vi "Initialize.vi"(7 "Serial Configuration":T1={"Baud Rate"=9600, "Parity"=0, "Data Bits"=8, "Stop Bits"=10, "Flow Control"=0} {"Flow Control" items=["None", "XON/XOFF", "RTS/CTS", "XON/XOFF & RTS/CTS", "DTR/DSR", "XON/XOFF & DTR/DSR"]; "Stop Bits" items=["1.0"=10, "1.5"=15, "2.0"=20]; "Data Bits" items=["7"=7, "8"=8]; "Parity" items=["None", "Odd", "Even", "Mark", "Space"]; "Baud Rate" items=["300"=300, "600"=600, "1200"=1200, "2400"=2400, "4800"=4800, "9600"=9600, "19200"=19200]}, 8 "error in":errorcluster, 9 "Reset":bool=TRUE, 10 "ID Query":bool=TRUE, 11 "VISA resource name":refnum<visa-resource-name>) -> (0 "error out":errorcluster, 3 "VISA resource name out":refnum<visa-resource-name>)   [LabVIEW 2020, in "IT-M3400.lvlib"]
doc: "Establishes communication with the instrument and optionally performs an instrument identification query and/or an instrument reset. It also places the instrument in a default state needed for other instrument driver operations. Therefore, call this VI before calling other instrument driver VIs for this instrument. Generally, you need to call the <b>Initialize</b> VI only once at the beginning of an application."
uses:
  IT-M3400.lvlib
panel:
  # "EDIT: Change control description to remove example text for buses not supported."
  # "EDIT: Serial settings must match those on the physical instrument.  Review user's manual to determine the correct Flow Control protocol for the instrument.  \"None\" is the least robust option for this setting, and could lead to unreliable data transmission."
  # "EDIT: If your instrument does not support ID query or Reset, remove the ID Query or Reset control from the front panel and delete the case structure with the ID Query or Reset code from the block diagram."
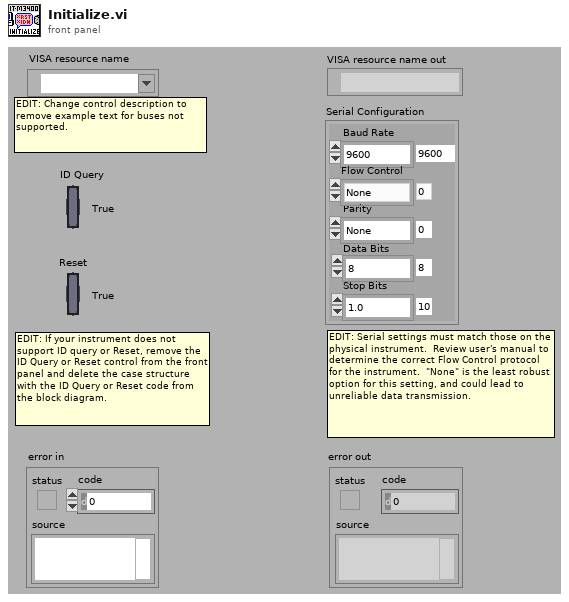
[diagram p1: front panel]
types:
  T1 = cluster{"Baud Rate":u32, "Parity":u16, "Data Bits":u16, "Stop Bits":u16, "Flow Control":u16}
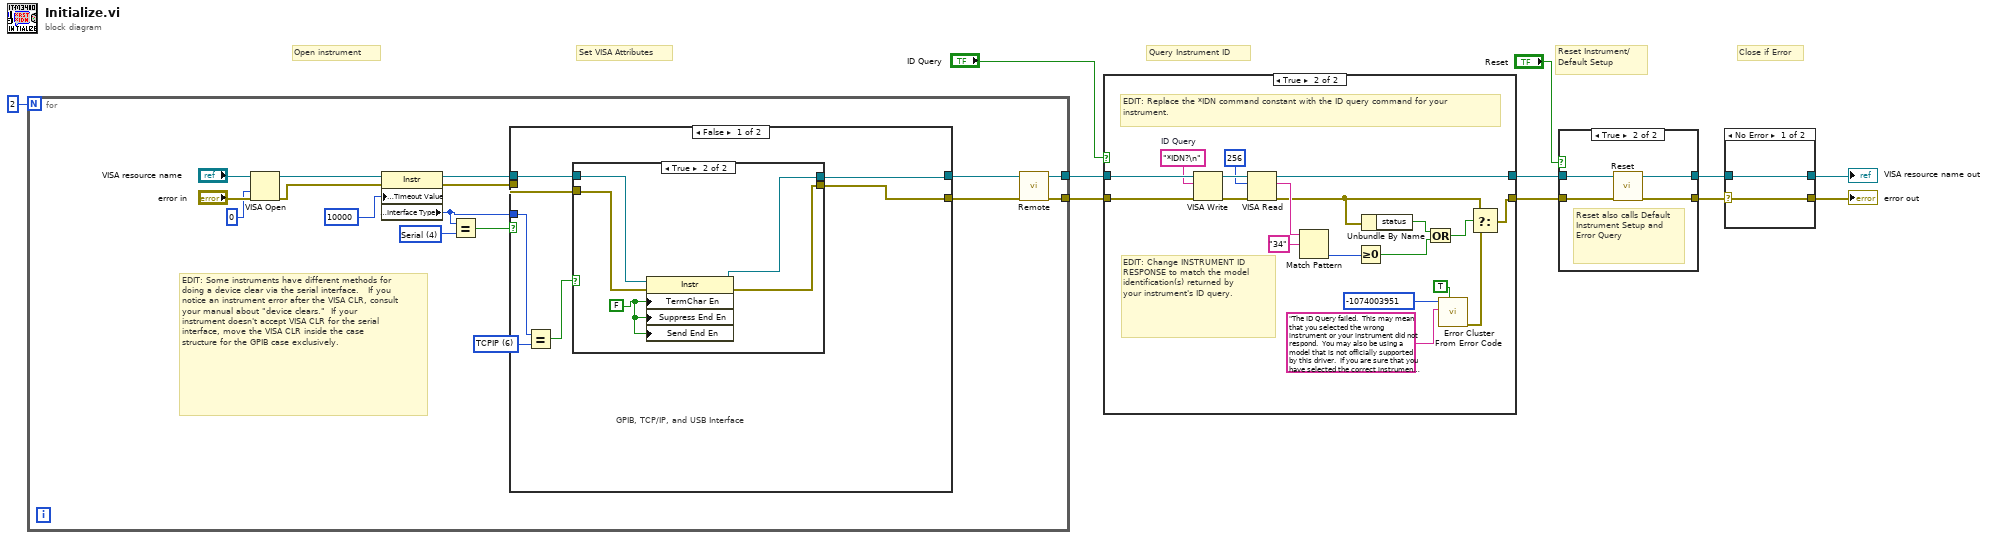
[diagram p0: block diagram]
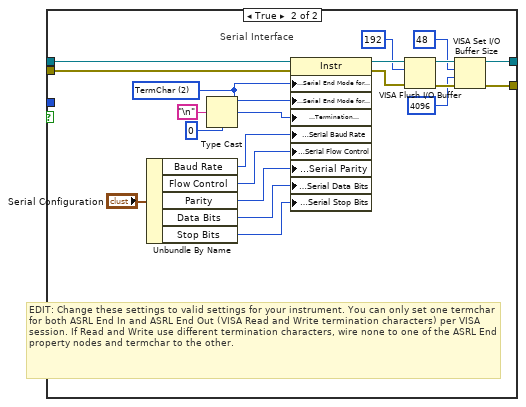
[diagram p3: hidden frame]
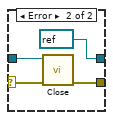
[diagram p4: hidden frame]
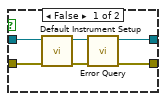
[diagram p5: hidden frame]
diagram:
  # "Set VISA Attributes"
  # "Close if Error"
  # "Query Instrument ID"
  # "Reset Instrument/\nDefault Setup"
  # "Open instrument"
  n1 = for {
    N: 2 -> [_]
    tunnel: [w16] -> w3
    tunnel: [w15] -> w2
    w21 = u16 4 items=["GPIB"=1, "VXI"=2, "GPIB-VXI"=3, "Serial"=4, "PXI"=5, "TCPIP"=6, "USB"=7] ("Interface Information:Interface Type")
    # "EDIT: Some instruments have different methods for doing a device clear via the serial interface.   If you notice an instrument error after the VISA CLR, consult your manual about \"device clears.\"  If your instrument doesn't accept VISA CLR for the serial interface, move the VISA CLR inside the case  structure for the GPIB case exclusively."
    n2 = VISA Open(access mode=u32 0, error in (no error)="error in", VISA resource name="VISA resource name") -> (VISA resource name=w13:refnum<visa-resource-name>, error out=w12:errorcluster)  [unwired: 2 in]
    n3 = property class="Instr"(reference=w13, error in=w12, "General Settings:Timeout Value"=u32 10000) -> (reference out=w23:refnum<visa-resource-name>, error out=w22:errorcluster, "Interface Information:Interface Type"=w19:u16)
    n4 = Equal?(x=w19, y=w21) -> (x = y?=w14:bool)
    n5 = case shown="False" w14 {
      tunnel: [w28 w58] -> w18
      tunnel: [w27 w55] -> w17
      tunnel: w23 -> [w30 w60]
      tunnel: w22 -> [w29 w61]
      tunnel: w19 -> [w31 _]
      frame False {
        w32 = u16 6 items=["GPIB"=1, "VXI"=2, "GPIB-VXI"=3, "Serial"=4, "PXI"=5, "TCPIP"=6, "USB"=7] ("Interface Information:Interface Type")
        # "GPIB, TCP/IP, and USB Interface"
        n6 = Equal?(x=w31, y=w32) -> (x = y?=w33:bool)
        n7 = case shown="True" w33 {
          tunnel: [w35 w40] -> w28
          tunnel: [w34 w39] -> w27
          tunnel: w30 -> [w35 w38]
          tunnel: w29 -> [w34 w37]
          frame False {
          }
          frame True {
            w36 = FALSE
            n8 = property class="Instr"(reference=w38, error in=w37, "TermChar En"=w36, "Suppress End En"=w36, "Send End En"=w36) -> (reference out=w40:refnum<visa-resource-name>, error out=w39:errorcluster)
          }
        }
      }
      frame True {
        w48 = u16 2 items=["None", "LastBit", "TermChar"] ("Serial Settings:Serial End Mode for Reads")
        # "EDIT: Change these settings to valid settings for your instrument. You can only set one termchar for both ASRL End In and ASRL End Out (VISA Read and Write termination characters) per VISA session. If Read and Write use different termination characters, wire none to one of the ASRL End property nodes and termchar to the other."
        # "Serial Interface"
        n9 = Unbundle By Name("Serial Configuration") -> ("Baud Rate"=w46:u32, "Flow Control"=w42:u16, "Parity"=w44:u16, "Data Bits"=w45:u16, "Stop Bits"=w41:u16)
        n10 = Type Cast(type=u8 0, x="\n" ("Line Feed Constant")) -> (*(type *) &x=w47:u8)
        n11 = property class="Instr"(reference=w60, error in=w61, "Serial Settings:Serial End Mode for Reads"=w48, "Serial Settings:Serial End Mode for Writes"=w48, "Message Based Settings:Termination Character"=w47, "Serial Settings:Serial Baud Rate"=w46, "Serial Settings:Serial Flow Control"=w42, "Serial Settings:Serial Parity"=w44, "Serial Settings:Serial Data Bits"=w45, "Serial Settings:Serial Stop Bits"=w41) -> (reference out=w54:refnum<visa-resource-name>, error out=w57:errorcluster)
        n12 = VISA Flush I/O Buffer(VISA resource name=w54, mask (16)=u16 192, error in (no error)=w57) -> (VISA resource name out=w59:refnum<visa-resource-name>, error out=w56:errorcluster)
        n13 = VISA Set I/O Buffer Size(VISA resource name=w59, mask (16)=u16 48, size (4096)=u32 4096 ("size (0)"), error in (no error)=w56) -> (VISA resource name out=w58:refnum<visa-resource-name>, error out=w55:errorcluster)
      }
    }
    n14 = call "Remote.vi"("error in"=w17, "VISA resource name"=w18) -> ("error out"=w15:errorcluster, "VISA resource name out"=w16:refnum<visa-resource-name>)  [unwired: 8 in]
  }
  n15 = case shown="True" "ID Query" {
    tunnel: [w62 w82] -> w10
    tunnel: [w63 w79] -> w11
    tunnel: w3 -> [w63 w80]
    tunnel: w2 -> [w62 w81]
    frame False {
    }
    frame True {
      w73 = "*IDN?\n"  # ID Query
      # "EDIT: Replace the *IDN command constant with the ID query command for your instrument."
      # "EDIT: Change INSTRUMENT ID RESPONSE to match the model identification(s) returned by your instrument's ID query."
      n16 = VISA Write(VISA resource name=w80, write buffer=w73, error in (no error)=w81) -> (VISA resource name out=w77:refnum<visa-resource-name>, error out=w76:errorcluster)  [unwired: 1 out]
      n17 = VISA Read(VISA resource name=w77, byte count=u32 256, error in (no error)=w76) -> (VISA resource name out=w79:refnum<visa-resource-name>, read buffer=w78:string, error out=w67:errorcluster)  [unwired: 1 out]
      n18 = Match Pattern(string=w78, regular expression="34") -> (offset past match=w68:i32)  [unwired: 1 in, 3 out]
      n19 = Greater Or Equal To 0?(x=w68) -> (x >= 0?=w65:bool)
      n20 = Unbundle By Name(w67) -> ("status"=w66:bool)
      n21 = Or(x=w66, y=w65) -> (x .or. y?=w64:bool)
      n22 = call <vilib>:"Error Cluster From Error Code.vi"("show call chain? (False)"=TRUE, "error message (\"\")"="The ID Query failed.  This may mean that you selected the wrong instrument or your instrument did not respond.  You may also be using a model that is not officially supported by this driver.  If you are sure that you have selected the correct instrument and it is responding, try disabling the ID Query." ("Source (VI Name)"), "error code (0)"=-1074003951 ("Code")) -> ("error out"=w72:errorcluster)  [unwired: 6 in]
      n23 = Select(t=w67, s=w64, f=w72) -> (s? t:f=w82:errorcluster)
    }
  }
  n24 = case shown="True" "Reset" {
    tunnel: w10 -> [w87 w89]
    tunnel: [w84 w92] -> w4
    tunnel: w11 -> [w88 w90]
    tunnel: [w85 w91] -> w5
    frame False {
      n25 = call "Default Instrument Setup.vi"("error in"=w87, "VISA resource name"=w88) -> ("error out"=w83:errorcluster, "VISA resource name out"=w86:refnum<visa-resource-name>)  [unwired: 8 in]
      n26 = call "Error Query.vi"("error in"=w83, "VISA resource name"=w86) -> ("error out"=w84:errorcluster, "VISA resource name out"=w85:refnum<visa-resource-name>)  [unwired: 6 in, 2 out]
    }
    frame True {
      # "Reset also calls Default Instrument Setup and Error Query"
      n27 = call "Reset.vi"("error in"=w89, "VISA resource name"=w90) -> ("error out"=w92:errorcluster, "VISA resource name out"=w91:refnum<visa-resource-name>)  [unwired: 8 in]
    }
  }
  n28 = case shown="No Error" w4 {
    selector: w4 -> [w93 w96]
    tunnel: w5 -> [w94 w97]
    tunnel: [w94 refnum<visa-resource-name> refnum ("VISA resource name out")] -> w7
    tunnel: [w93 w98] -> w6
    frame No Error {
    }
    frame Error {
      n29 = call "Close.vi"("error in"=w96, "VISA resource name"=w97) -> ("error out"=w98:errorcluster)  [unwired: 9 in]
    }
  }
  "VISA resource name out" <- w7
  "error out" <- w6
